vi "Configure Module.vi"(8 "error in (no error)":errorcluster, 10 "IOV ref in":variant, 11 "9214 in":refnum<class "9214.lvclass">) -> (0 "error out":errorcluster, 2 "IOV ref out":variant, 3 "9214 out":refnum<class "9214.lvclass">)   [LabVIEW 2017, in "Modules.lvlib" / "9214.lvclass"]
uses:
  9214.lvclass
  <resource>/objmgr/cRIO.rc
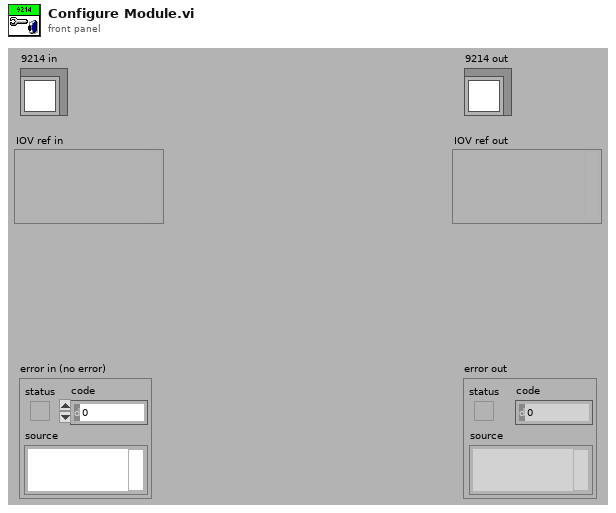
[diagram p1: front panel]
types:
  T1 = typedef "Modules.lvlib/9213.lvclass/Conversion Time.ctl" = u16
  T2 = typedef "Modules.lvlib/9213.lvclass/Measurement Units.ctl" = u8
  T3 = typedef "Modules.lvlib/9213.lvclass/Thermocouple Type.ctl" = u8
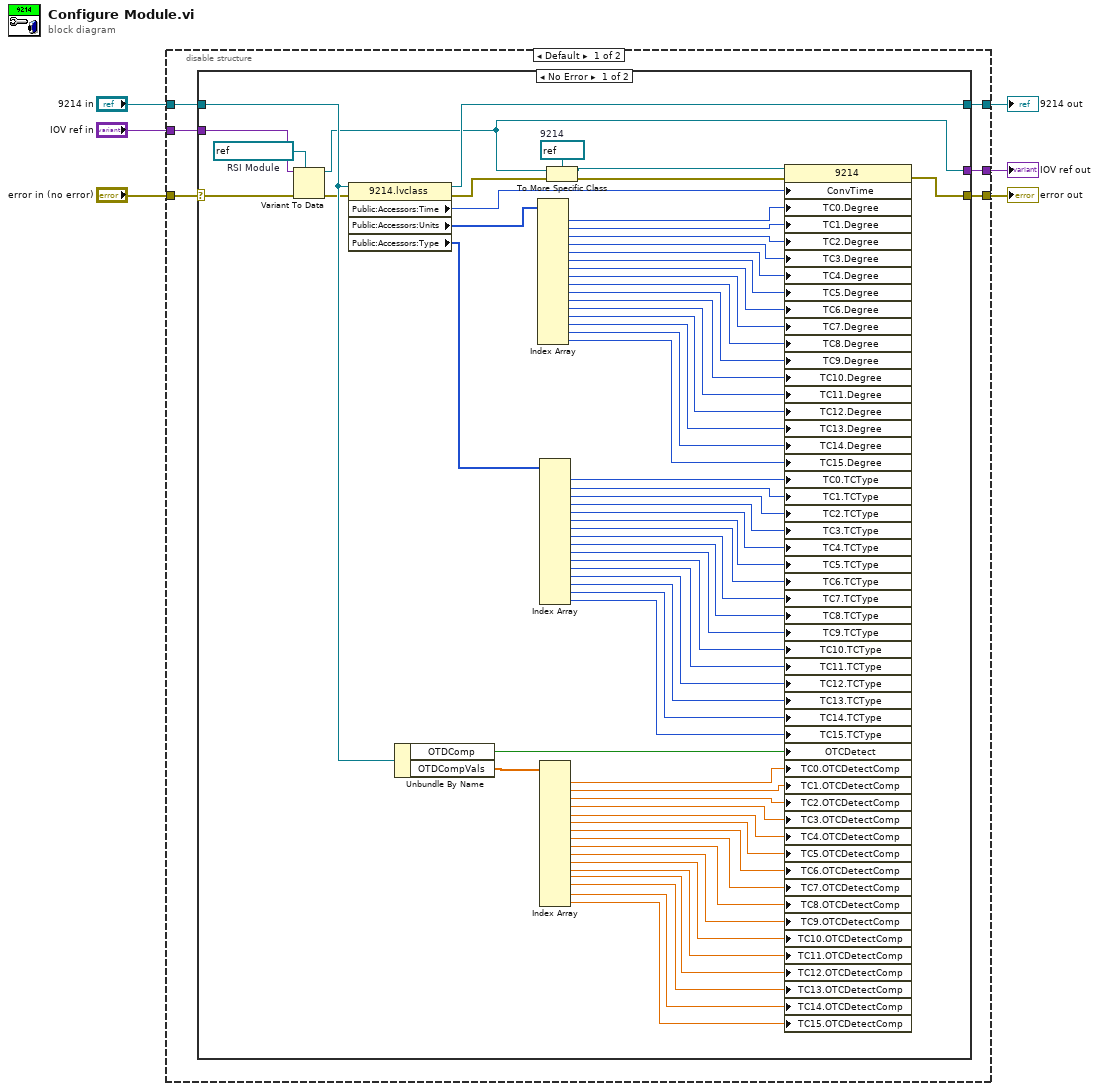
[diagram p0: block diagram]
diagram:
  n1 = disable-structure shown="Default" {
    disable-tunnel: "error in (no error)" -> [w12 w83]
    disable-tunnel: [w11 w83] -> w5
    disable-tunnel: "9214 in" -> [w10 w81]
    disable-tunnel: [w9 w81] -> w3
    disable-tunnel: "IOV ref in" -> [w8 w82]
    disable-tunnel: [w7 w82] -> w1
    frame condition #0 (active) {
      n2 = case shown="No Error" w12 {
        selector: w12 -> [w23 w80]
        tunnel: [w77 w80] -> w11
        tunnel: [w20 w79] -> w9
        tunnel: w10 -> [w22 w79]
        tunnel: w8 -> [w15 w78]
        tunnel: [w14 w78] -> w7
        frame No Error {
          w13 = refnum<k21> refnum  # RSI Module
          w76 = refnum<k21> refnum  # 9214
          n3 = Variant To Data(error in=w23, type=w13, Variant=w15) -> (data=w14:refnum<k21>, error out=w16:errorcluster)
          n4 = property class="9214.lvclass"(reference=w22, error in=w16) -> (reference out=w20:refnum<class "9214.lvclass">, error out=w21:errorcluster, "Public:Accessors:Time"=w17:T1, "Public:Accessors:Units"=w18:T2[], "Public:Accessors:Type"=w19:T3[])
          n5 = Unbundle By Name(w22) -> ("OTDComp"=w41:bool, "OTDCompVals"=w40:dbl[])
          n6 = Index Array(array=w18) -> (element #1=w73:T2, element #2=w72:T2, element #3=w71:T2, element #4=w70:T2, element #5=w69:T2, element #6=w68:T2, element #7=w67:T2, element #8=w66:T2, element #9=w65:T2, element #10=w64:T2, element #11=w63:T2, element #12=w62:T2, element #13=w61:T2, element #14=w60:T2, element #15=w59:T2, element #16=w58:T2)  [unwired: 16 in]
          n7 = Index Array(array=w19) -> (element #1=w57:T3, element #2=w56:T3, element #3=w55:T3, element #4=w54:T3, element #5=w53:T3, element #6=w52:T3, element #7=w51:T3, element #8=w50:T3, element #9=w49:T3, element #10=w48:T3, element #11=w47:T3, element #12=w46:T3, element #13=w45:T3, element #14=w44:T3, element #15=w43:T3, element #16=w42:T3)  [unwired: 16 in]
          n8 = Index Array(array=w40) -> (element #1=w39:dbl, element #2=w38:dbl, element #3=w37:dbl, element #4=w36:dbl, element #5=w35:dbl, element #6=w34:dbl, element #7=w33:dbl, element #8=w32:dbl, element #9=w31:dbl, element #10=w30:dbl, element #11=w29:dbl, element #12=w28:dbl, element #13=w27:dbl, element #14=w26:dbl, element #15=w25:dbl, element #16=w24:dbl)  [unwired: 16 in]
          n9 = To More Specific Class(target class=w76, reference=w14, error in=w21) -> (specific class reference=w75:refnum<k21>, error out=w74:errorcluster)
          n10 = property class="9214"(reference=w75, error in=w74, "ConvTime"=w17, "TC0.Degree"=w73, "TC1.Degree"=w72, "TC2.Degree"=w71, "TC3.Degree"=w70, "TC4.Degree"=w69, "TC5.Degree"=w68, "TC6.Degree"=w67, "TC7.Degree"=w66, "TC8.Degree"=w65, "TC9.Degree"=w64, "TC10.Degree"=w63, "TC11.Degree"=w62, "TC12.Degree"=w61, "TC13.Degree"=w60, "TC14.Degree"=w59, "TC15.Degree"=w58, "TC0.TCType"=w57, "TC1.TCType"=w56, "TC2.TCType"=w55, "TC3.TCType"=w54, "TC4.TCType"=w53, "TC5.TCType"=w52, "TC6.TCType"=w51, "TC7.TCType"=w50, "TC8.TCType"=w49, "TC9.TCType"=w48, "TC10.TCType"=w47, "TC11.TCType"=w46, "TC12.TCType"=w45, "TC13.TCType"=w44, "TC14.TCType"=w43, "TC15.TCType"=w42, "OTCDetect"=w41, "TC0.OTCDetectComp"=w39, "TC1.OTCDetectComp"=w38, "TC2.OTCDetectComp"=w37, "TC3.OTCDetectComp"=w36, "TC4.OTCDetectComp"=w35, "TC5.OTCDetectComp"=w34, "TC6.OTCDetectComp"=w33, "TC7.OTCDetectComp"=w32, "TC8.OTCDetectComp"=w31, "TC9.OTCDetectComp"=w30, "TC10.OTCDetectComp"=w29, "TC11.OTCDetectComp"=w28, "TC12.OTCDetectComp"=w27, "TC13.OTCDetectComp"=w26, "TC14.OTCDetectComp"=w25, "TC15.OTCDetectComp"=w24) -> (error out=w77:errorcluster)  [unwired: 1 out]
        }
        frame Error {
        }
      }
    }
    frame condition #1 {
    }
  }
  "error out" <- w5
  "9214 out" <- w3
  "IOV ref out" <- w1
